vi "OSICS_Closeport.vi"(8 "error in":errorcluster, 11 "VISA IN":refnum<visa-resource-name>) -> (0 "error out":errorcluster)   [LabVIEW 2014, in "OSICS_LIB.lvlib"]
doc: "This VI closes the data communication."
uses:
  OSICS_LIB.lvlib
  <vilib>/Instr/_visa.llb/VISA GPIB Control REN Mode.ctl
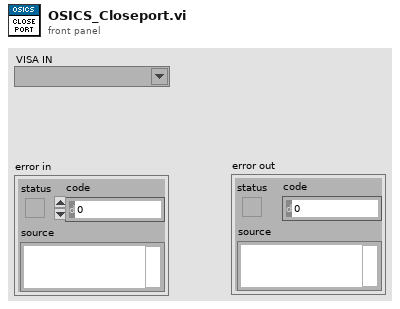
[diagram p1: front panel]
types:
  T1 = typedef "VISA GPIB Control REN Mode.ctl" = u16
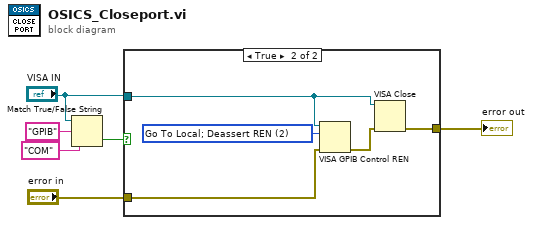
[diagram p0: block diagram]
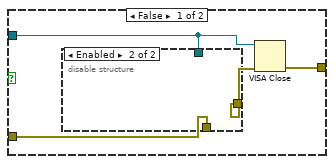
[diagram p2: hidden frame]
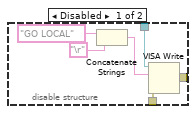
[diagram p3: hidden frame]
diagram:
  n1 = Match True/False String(2:"COM" ("false string"), 3:"GPIB" ("true string"), 4:"VISA IN") -> (0:w5:bool)  [unwired: 1 out]
  n2 = case shown="True" w5 {
    tunnel: "VISA IN" -> [w8 w20]
    tunnel: "error in" -> [w9 w19]
    tunnel: [w10 w18] -> w1
    frame False {
      n3 = disable-structure shown="Enabled" {
        disable-tunnel: w9 -> [w14 _]
        disable-tunnel: w8 -> [w13 _]
        disable-tunnel: [w11 _] -> w7
        frame Disabled {
          n4 = Concatenate Strings("GO LOCAL" ("string"), "\r") -> (w12:string)
          n5 = VISA Write(VISA resource name=w13, write buffer=w12, error in (no error)=w14) -> (error out=w11:errorcluster)  [unwired: 2 out]
        }
        frame Enabled {
        }
      }
      n6 = VISA Close(VISA resource name=w8, error in (no error)=w7) -> (error out=w10:errorcluster)
    }
    frame True {
      w17 = T1 2 items=["Deassert REN", "Assert REN", "Go To Local; Deassert REN ", "Assert REN; Address Device", "Local Lockout (Addressed Devices)", "Local Lockout (This Device)", "Go To Local"] ("Mode")
      n7 = VISA GPIB Control REN(8:w19, 10:w17, 11:w20) -> (0:w21:errorcluster)  [unwired: 1 out]
      n8 = VISA Close(VISA resource name=w20, error in (no error)=w21) -> (error out=w18:errorcluster)
    }
  }
  "error out" <- w1
